vi "Slope Calibration.vi"(0 "Voltage":dynamicdata(waveform), 5 "Slope":dynamicdata(waveform), 7 "Intercept":dynamicdata(waveform), 11 "error in (no error)":errorcluster) -> (4 "Result":dynamicdata(waveform), 15 "error out":errorcluster)   [LabVIEW 2020, in "CollectionSupport.lvlib"]
uses:
  CollectionSupport.lvlib
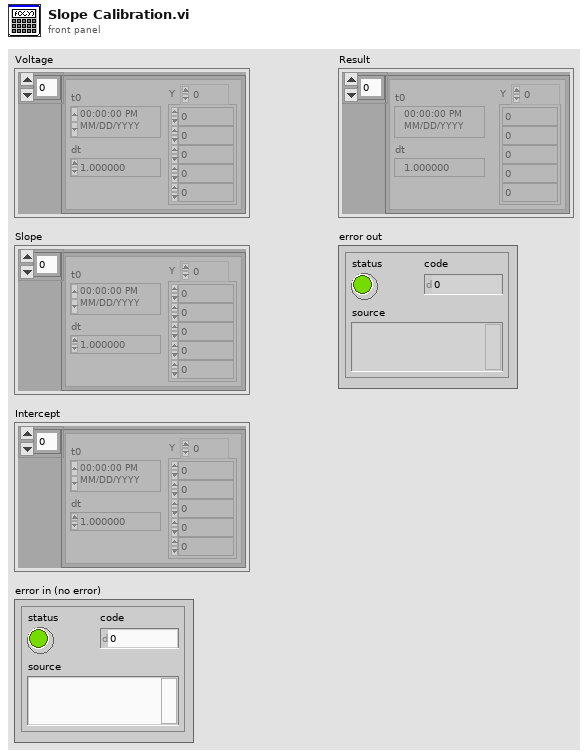
[diagram p1: front panel]
types:
  T1 = enum32{"X1", "X2", "X3", "X4", "X5", "X6", "X7", "X8"}
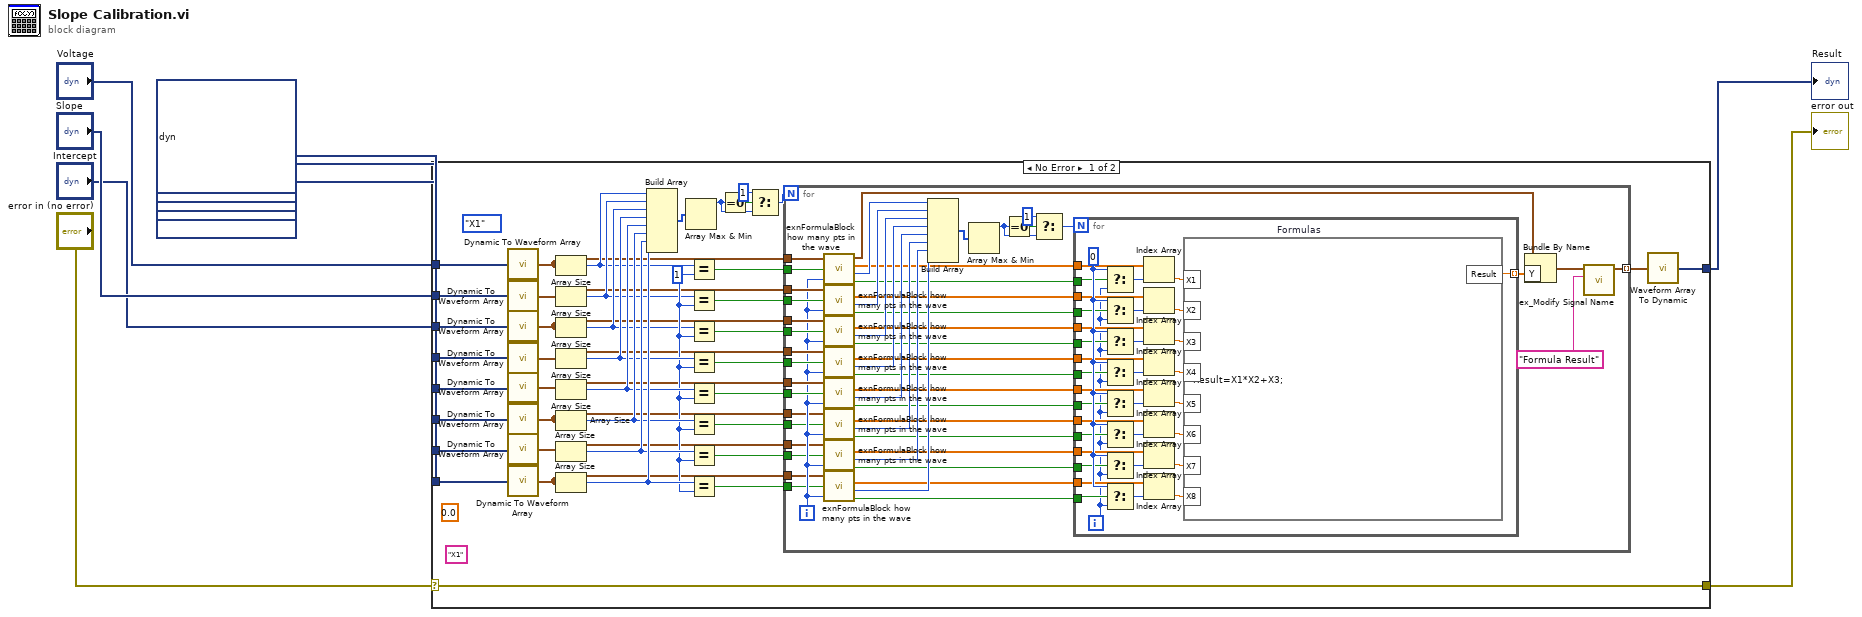
[diagram p0: block diagram]
diagram:
  n1 = case shown="No Error" "error in (no error)" {
    selector: "error in (no error)" -> [w12 w139]
    tunnel: [w20 _] -> w7
    tunnel: [w12 w139] -> w6
    tunnel: dynamicdata [] ("X5") -> [w22 _]
    tunnel: dynamicdata [] ("X4") -> [w23 _]
    tunnel: "Intercept" -> [w24 _]
    tunnel: "Slope" -> [w25 _]
    tunnel: "Voltage" -> [w27 _]
    tunnel: dynamicdata [] ("X8") -> [w29 _]
    tunnel: dynamicdata [] ("X7") -> [w26 _]
    tunnel: dynamicdata [] ("X6") -> [w21 _]
    frame No Error {
      (unwired) T1."X1" ("Tab Control")
      (unwired) 0.0 ("numinputs")
      (unwired) "X1" ("Formula Output")
      w46 = u8 1 ("y")
      n2 = call <vilib>:"Dynamic To Waveform Array.vi"("Input"=w27) -> ("Output"=w28:waveform(dbl)[])  [unwired: 4 in]
      n3 = call <vilib>:"Dynamic To Waveform Array.vi"("Input"=w25) -> ("Output"=w19:waveform(dbl)[])  [unwired: 4 in]
      n4 = call <vilib>:"Dynamic To Waveform Array.vi"("Input"=w24) -> ("Output"=w18:waveform(dbl)[])  [unwired: 4 in]
      n5 = call <vilib>:"Dynamic To Waveform Array.vi"("Input"=w23) -> ("Output"=w17:waveform(dbl)[])  [unwired: 4 in]
      n6 = call <vilib>:"Dynamic To Waveform Array.vi"("Input"=w22) -> ("Output"=w16:waveform(dbl)[])  [unwired: 4 in]
      n7 = call <vilib>:"Dynamic To Waveform Array.vi"("Input"=w21) -> ("Output"=w15:waveform(dbl)[])  [unwired: 4 in]
      n8 = call <vilib>:"Dynamic To Waveform Array.vi"("Input"=w26) -> ("Output"=w14:waveform(dbl)[])  [unwired: 4 in]
      n9 = call <vilib>:"Dynamic To Waveform Array.vi"("Input"=w29) -> ("Output"=w13:waveform(dbl)[])  [unwired: 4 in]
      n10 = Array Size(array=w28) -> (size(s)=w43:i32)
      n11 = Array Size(array=w19) -> (size(s)=w44:i32)
      n12 = Array Size(array=w18) -> (size(s)=w45:i32)
      n13 = Array Size(array=w17) -> (size(s)=w47:i32)
      n14 = Array Size(array=w16) -> (size(s)=w48:i32)
      n15 = Array Size(array=w15) -> (size(s)=w49:i32)
      n16 = Array Size(array=w14) -> (size(s)=w50:i32)
      n17 = Array Size(array=w13) -> (size(s)=w51:i32)
      n18 = Build Array(w43, w44, w45, w47, w48, w49, w50, w51) -> (w42:i32[])
      n19 = Array Max & Min(array=w42) -> (max value=w32:i32)  [unwired: 3 out]
      n20 = Equal?(x=w43, y=w46) -> (x = y?=w41:bool)
      n21 = Equal?(x=w44, y=w46) -> (x = y?=w40:bool)
      n22 = Equal?(x=w45, y=w46) -> (x = y?=w39:bool)
      n23 = Equal?(x=w47, y=w46) -> (x = y?=w38:bool)
      n24 = Equal?(x=w48, y=w46) -> (x = y?=w37:bool)
      n25 = Equal?(x=w49, y=w46) -> (x = y?=w36:bool)
      n26 = Equal?(x=w50, y=w46) -> (x = y?=w35:bool)
      n27 = Equal?(x=w51, y=w46) -> (x = y?=w34:bool)
      n28 = Equal To 0?(x=w32) -> (x = 0?=w33:bool)
      n29 = Select(t=1, s=w33, f=w32) -> (s? t:f=w30:i32)
      n30 = for {
        N: w30 -> [_]
        tunnel: [w54] -> w52 mode=indexing
        tunnel: w41 -> [w100]
        tunnel: w40 -> [w97]
        tunnel: w39 -> [w94]
        tunnel: w38 -> [w91]
        tunnel: w37 -> [w87]
        tunnel: w36 -> [w82]
        tunnel: w35 -> [w81]
        tunnel: w34 -> [w80]
        tunnel: w28 -> [w98]
        tunnel: w19 -> [w95]
        tunnel: w18 -> [w92]
        tunnel: w17 -> [w89]
        tunnel: w16 -> [w88]
        tunnel: w15 -> [w83]
        tunnel: w14 -> [w84]
        tunnel: w13 -> [w85]
        i -> [w86]
        n31 = call <vilib>:"exnFormulaBlock how many pts in the wave.vi"("Array"=w98, "Boolean"=w100, "Iteration"=w86) -> ("Waveform"=w101:waveform(dbl), "Y"=w75:dbl[], "size(s)"=w99:i32, "x = y?"=w74:bool)
        n32 = call <vilib>:"exnFormulaBlock how many pts in the wave.vi"("Array"=w95, "Boolean"=w97, "Iteration"=w86) -> ("Y"=w73:dbl[], "size(s)"=w96:i32, "x = y?"=w72:bool)  [unwired: 1 out]
        n33 = call <vilib>:"exnFormulaBlock how many pts in the wave.vi"("Array"=w92, "Boolean"=w94, "Iteration"=w86) -> ("Y"=w71:dbl[], "size(s)"=w93:i32, "x = y?"=w70:bool)  [unwired: 1 out]
        n34 = call <vilib>:"exnFormulaBlock how many pts in the wave.vi"("Array"=w89, "Boolean"=w91, "Iteration"=w86) -> ("Y"=w69:dbl[], "size(s)"=w90:i32, "x = y?"=w63:bool)  [unwired: 1 out]
        n35 = call <vilib>:"exnFormulaBlock how many pts in the wave.vi"("Array"=w88, "Boolean"=w87, "Iteration"=w86) -> ("Y"=w68:dbl[], "size(s)"=w79:i32, "x = y?"=w67:bool)  [unwired: 1 out]
        n36 = call <vilib>:"exnFormulaBlock how many pts in the wave.vi"("Array"=w83, "Boolean"=w82, "Iteration"=w86) -> ("Y"=w66:dbl[], "size(s)"=w78:i32, "x = y?"=w62:bool)  [unwired: 1 out]
        n37 = call <vilib>:"exnFormulaBlock how many pts in the wave.vi"("Array"=w84, "Boolean"=w81, "Iteration"=w86) -> ("Y"=w65:dbl[], "size(s)"=w77:i32, "x = y?"=w61:bool)  [unwired: 1 out]
        n38 = call <vilib>:"exnFormulaBlock how many pts in the wave.vi"("Array"=w85, "Boolean"=w80, "Iteration"=w86) -> ("Y"=w64:dbl[], "size(s)"=w76:i32, "x = y?"=w60:bool)  [unwired: 1 out]
        n39 = Build Array(w99, w96, w93, w90, w79, w78, w77, w76) -> (w102:i32[])
        n40 = Array Max & Min(array=w102) -> (max value=w57:i32)  [unwired: 3 out]
        n41 = Equal To 0?(x=w57) -> (x = 0?=w59:bool)
        n42 = Select(t=u8 1, s=w59, f=w57) -> (s? t:f=w56:i32)
        n43 = for {
          N: w56 -> [_]
          tunnel: [w138] -> w103 mode=indexing
          tunnel: w75 -> [w127]
          tunnel: w74 -> [w126]
          tunnel: w73 -> [w125]
          tunnel: w72 -> [w124]
          tunnel: w71 -> [w123]
          tunnel: w70 -> [w122]
          tunnel: w69 -> [w121]
          tunnel: w68 -> [w120]
          tunnel: w67 -> [w119]
          tunnel: w66 -> [w118]
          tunnel: w65 -> [w117]
          tunnel: w64 -> [w116]
          tunnel: w63 -> [w115]
          tunnel: w62 -> [w114]
          tunnel: w61 -> [w113]
          tunnel: w60 -> [w105]
          i -> [w104]
          w137 = 0 ("t")
          n44 = Select(t=w137, s=w126, f=w104) -> (s? t:f=w133:i32)
          n45 = Select(t=w137, s=w124, f=w104) -> (s? t:f=w132:i32)
          n46 = Select(t=w137, s=w122, f=w104) -> (s? t:f=w131:i32)
          n47 = Select(t=w137, s=w115, f=w104) -> (s? t:f=w130:i32)
          n48 = Select(t=w137, s=w119, f=w104) -> (s? t:f=w129:i32)
          n49 = Select(t=w137, s=w114, f=w104) -> (s? t:f=w134:i32)
          n50 = Select(t=w137, s=w113, f=w104) -> (s? t:f=w135:i32)
          n51 = Select(t=w137, s=w105, f=w104) -> (s? t:f=w136:i32)
          n52 = Index Array(array=w127, index=w133) -> (element=w128:dbl)
          n53 = Index Array(array=w125, index=w132) -> (element=w112:dbl)
          n54 = Index Array(array=w123, index=w131) -> (element=w111:dbl)
          n55 = Index Array(array=w121, index=w130) -> (element=w110:dbl)
          n56 = Index Array(array=w120, index=w129) -> (element=w109:dbl)
          n57 = Index Array(array=w118, index=w134) -> (element=w108:dbl)
          n58 = Index Array(array=w117, index=w135) -> (element=w107:dbl)
          n59 = Index Array(array=w116, index=w136) -> (element=w106:dbl)
          n60 = formula code="Result=X1*X2+X3;" "Formulas"("X1"=w128, "X2"=w112, "X3"=w111, "X4"=w110, "X5"=w109, "X6"=w108, "X7"=w107, "X8"=w106) -> ("Result"=w138:dbl)
        }
        n61 = Bundle By Name(cluster=w101, "Y"=w103) -> (w55:waveform(dbl))
        n62 = call <vilib>:"ex_Modify Signal Name.vi"("Name Modifier"="Formula Result", "waveform in"=w55) -> ("waveform out"=w54:waveform(dbl))  [unwired: 8 in, 1 out]
      }
      n63 = call <vilib>:"Waveform Array To Dynamic.vi"("Input"=w52) -> ("Output"=w20:dynamicdata)  [unwired: 4 in]
    }
    frame Error {
    }
  }
  "Result" <- w7
  "error out" <- w6
